vi "Set Scroll Bar State.vi"(8 "错误输入":cluster{"状态":bool, "代码":i32, "源":string}, 10 "滚动条可见（始终打开）":T1(ring), 11 "窗格引用输入":refnum<vi>) -> (0 "错误输出":cluster{"状态":bool, "代码":i32, "源":string}, 3 "窗格引用输出":refnum<vi>)   [LabVIEW 2012]
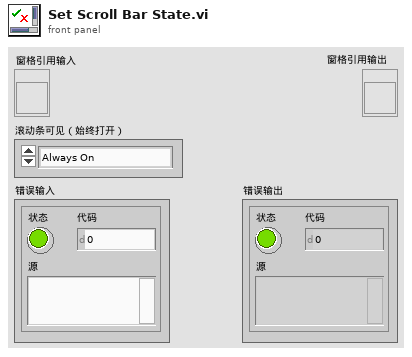
[diagram p1: front panel]
types:
  T1 = enum16{"Always On", "Always Off", "Off While Running"}
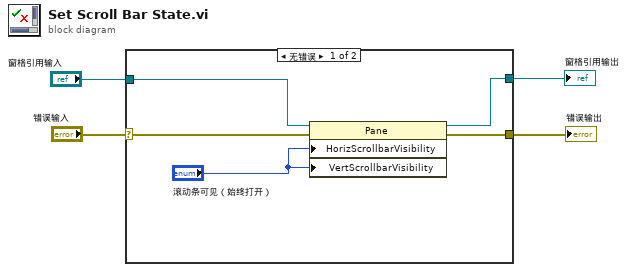
[diagram p0: block diagram]
diagram:
  n1 = case shown="无错误" "错误输入" {
    selector: "错误输入" -> [w8 w11]
    tunnel: [w7 w11] -> w3
    tunnel: "窗格引用输入" -> [w9 w10]
    tunnel: [w6 w10] -> w1
    frame No Error {
      n2 = property on="属性节点" class="Pane"(reference=w9, error in=w8, "HorizScrollbarVisibility"="滚动条可见（始终打开）", "VertScrollbarVisibility"="滚动条可见（始终打开）") -> (reference out=w6:refnum<vi>, error out=w7:errorcluster)
    }
    frame Error {
    }
  }
  "错误输出" <- w3
  "窗格引用输出" <- w1
